vi "DB_Action-UpdateModule.vi"(8 "error in":errorcluster, 10 "UUT输入":T1) -> (0 "error out":errorcluster)   [LabVIEW 2015, in "Settings-Style.lvlib"]
uses:
  Settings-Style.lvlib
  1_Ctl/DB_UUT.ctl
  1_ctl/Ctl-Color.ctl
panel:
  out "Result":string caption="结果"
  # "Style Settings"
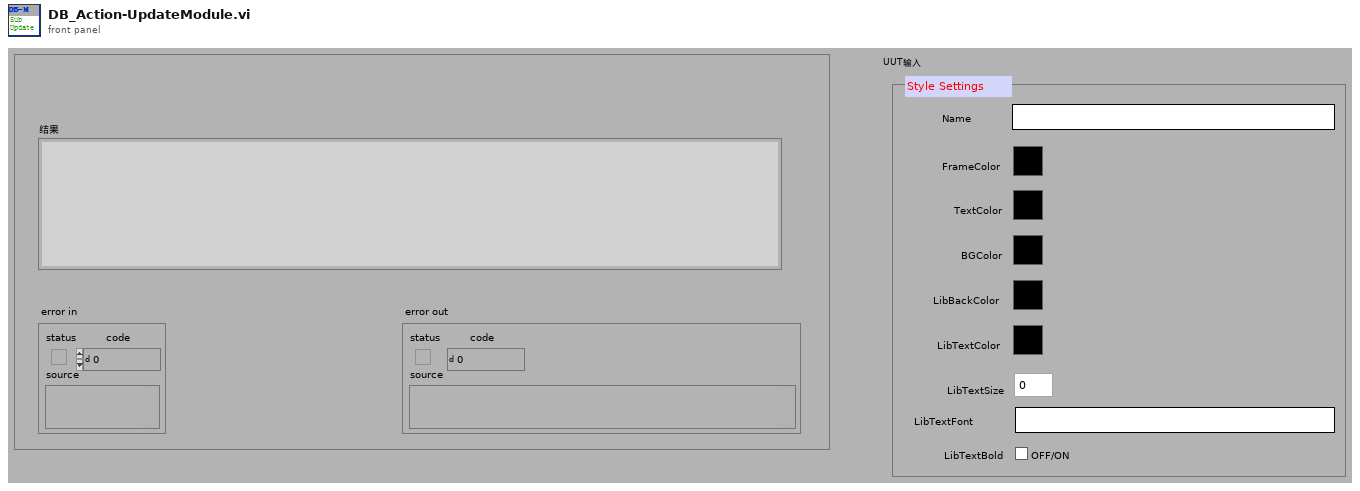
[diagram p1: front panel]
types:
  T1 = typedef "Settings-Style.lvlib/DB_UUT.ctl" = cluster{"Name":string, "FrameColor":T2, "TextColor":T2, "BGColor":T2, "LibBackColor":T2, "LibTextColor":T2, "LibTextSize":u32, "LibTextFont":string, "LibTextBold":bool}
  T2 = typedef "Ctl-Color.ctl" = u32
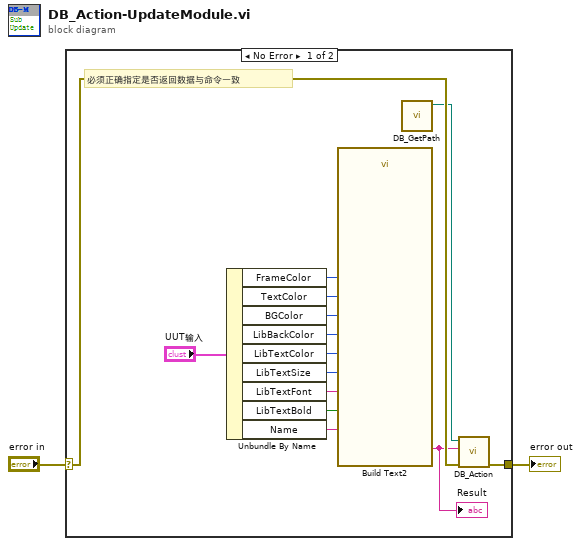
[diagram p0: block diagram]
diagram:
  n1 = case shown="No Error" "error in" {
    selector: "error in" -> [w15 w17]
    tunnel: [w16 w17] -> w2
    frame No Error {
      # "必须正确指定是否返回数据与命令一致"
      n2 = Unbundle By Name("UUT输入") -> ("FrameColor"=w12:T2, "TextColor"=w11:T2, "BGColor"=w10:T2, "LibBackColor"=w9:T2, "LibTextColor"=w8:T2, "LibTextSize"=w7:u32, "LibTextFont"=w6:string, "LibTextBold"=w5:bool, "Name"=w4:string)
      n3 = call "Build Text2"("FrameColor"=w12, "TextColor"=w11, "BGColor"=w10, "LibBackColor"=w9, "LibTextColor"=w8, "LibTextSize"=w7, "LibTextFont"=w6, "LibTextBold"=w5, "Name"=w4) -> ("Result"=w3:string)  [unwired: 17 in, 1 out]
      "Result" <- w3
      n4 = call "DB_GetPath.vi"() -> ("appended path"=w14:path)  [unwired: 11 in]
      n5 = call "DB_Action.vi"("error in"=w15, "Command Text"=w3, "路径"=w14) -> ("error out"=w16:errorcluster)  [unwired: 7 in, 1 out]
    }
    frame Error {
    }
  }
  "error out" <- w2
